vi "Burning DeQueue.vi"(8 "error in (no error) 2":errorcluster) -> (0 "error out":errorcluster, 2 "element":T1=enum."Main", 3 "queue out":refnum<queue>)   [LabVIEW 2022 SP3]
uses:
  Type Def/Burning States.ctl
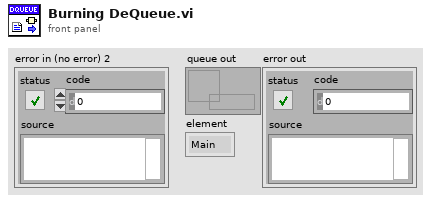
[diagram p1: front panel]
types:
  T1 = typedef "Burning States.ctl" = enum16{"Open Ports", "Close Ports", "Main", "Settings", "Voltaje", "Probe", "Lenguaje", "Callibration", "Exit", "Voltage Test", "Test 2", "End test"}
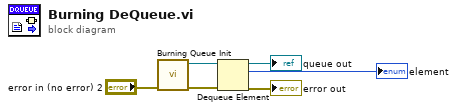
[diagram p0: block diagram]
diagram:
  n1 = call "Burning Queue Init.vi"("error in (no error) 2"="error in (no error) 2") -> ("error out 2"=w5:errorcluster, "queue out 2"=w6:refnum<queue>)  [unwired: 9 in]
  n2 = Dequeue Element(queue=w6, error in (no error)=w5) -> (queue out=→"queue out":refnum<queue>, element=→"element":T1, error out=→"error out":errorcluster)  [unwired: 1 in, 1 out]
